vi "CheesyDrive2016Ported.vi"(9 "Is Quick Turn":bool, 10 "Wheel":dbl(slide) scale=-1.0..1.0, 11 "Throttle":dbl(slide) scale=-1.0..1.0) -> (2 "RightOutput":dbl, 3 "LeftOutput":dbl)   [LabVIEW 2018]
panel:
  in  "Alpha":dbl
  in  "Wheel Deadband":dbl
  in  "Throttle Deadband":dbl
  in  "TurnSensitivity":dbl
  # "Direct Port to Labveiw from https://github.com/Team254/FRC-2016-Public/blob/master/src/com/team254/frc2016/CheesyDriveHelper.java"
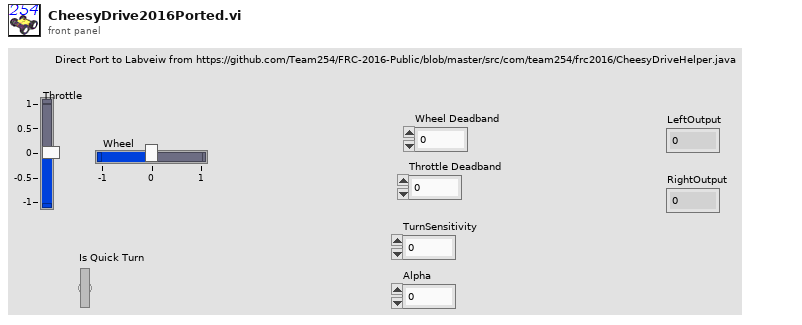
[diagram p1: front panel]
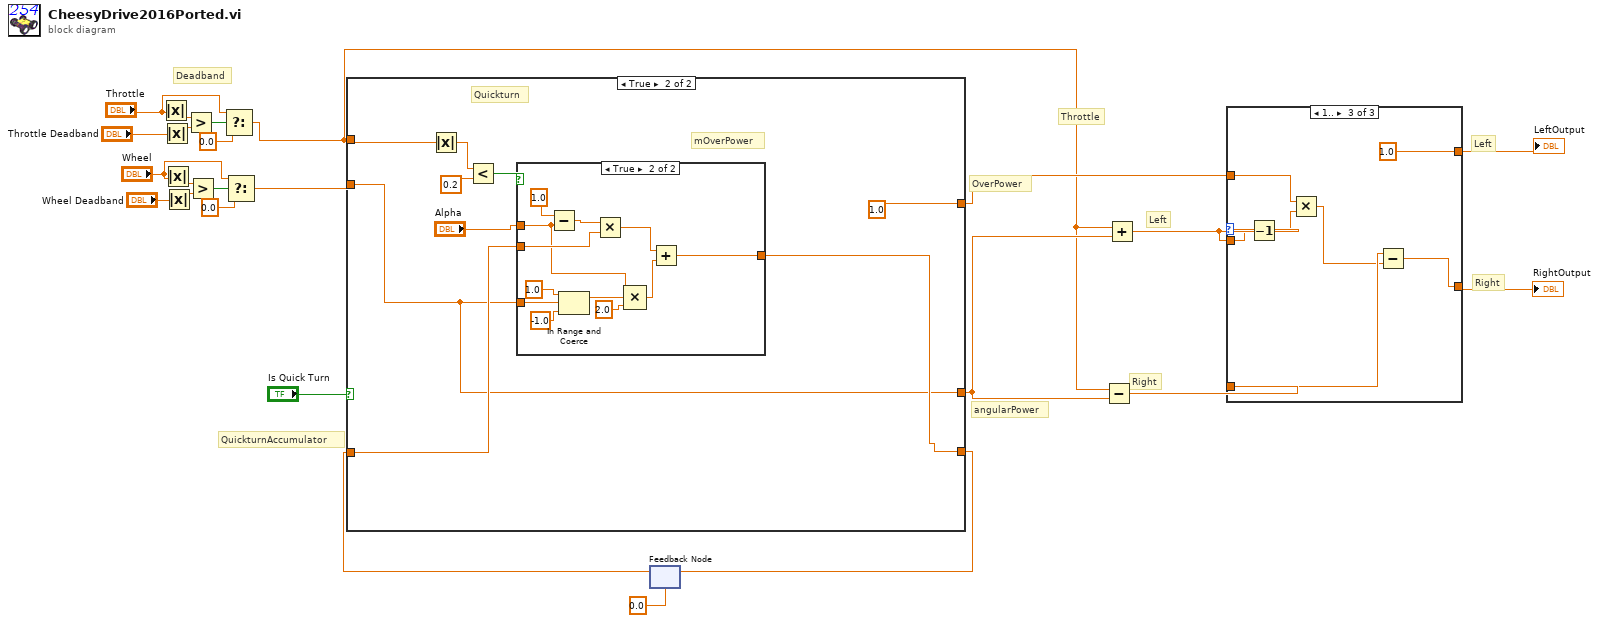
[diagram p0: block diagram]
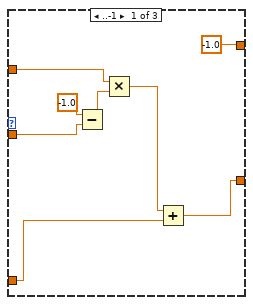
[diagram p2: hidden frame]
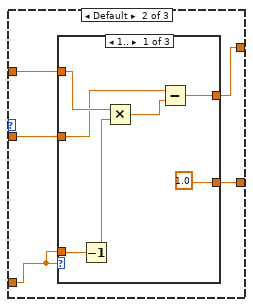
[diagram p3: hidden frame]
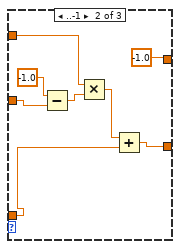
[diagram p4: hidden frame]
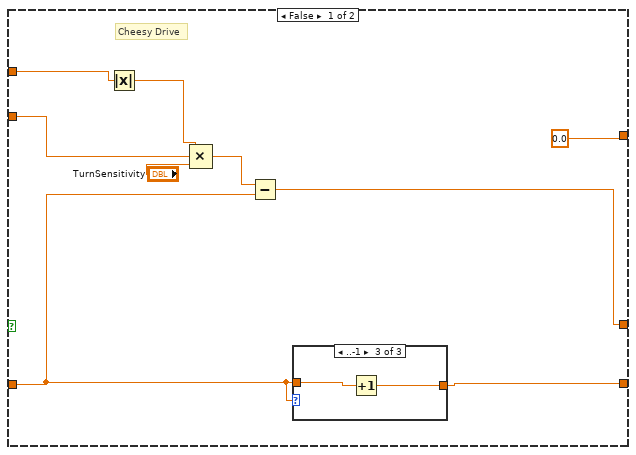
[diagram p6: hidden frame]
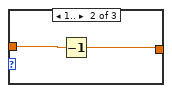
[diagram p8: hidden frame]
diagram:
  # "Deadband"
  # "Right"
  # "Left"
  # "Throttle"
  # "Left"
  # "Right"
  # "QuickturnAccumulator"
  # "angularPower"
  # "OverPower"
  n1 = Absolute Value(x="Throttle") -> (abs(x)=w15:dbl)
  n2 = Absolute Value(x="Throttle Deadband") -> (abs(x)=w14:dbl)
  n3 = Absolute Value(x="Wheel") -> (abs(x)=w10:dbl)
  n4 = Absolute Value(x="Wheel Deadband") -> (abs(x)=w11:dbl)
  n5 = Greater?(x=w15, y=w14) -> (0:w16:bool)
  n6 = Greater?(x=w10, y=w11) -> (0:w9:bool)
  n7 = Select(t="Throttle", s=w16, f=0.0) -> (s? t:f=w7:dbl)
  n8 = Select(t="Wheel", s=w9, f=0.0) -> (s? t:f=w8:dbl)
  n9 = feedback #1(0.0) -> (w22:dbl)
  n10 = case shown="True" "Is Quick Turn" {
    tunnel: w7 -> [w33 w47]
    tunnel: w8 -> [w31 w40]
    tunnel: [w26 w42] -> w23
    tunnel: w22 -> [w27 w43]
    tunnel: [0.0 1.0] -> w19
    tunnel: [w29 w40] -> w20
    frame False {
      # "Cheesy Drive"
      n11 = Absolute Value(x=w33) -> (abs(x)=w32:dbl)
      n12 = Compound Arithmetic op=MULTIPLY(w32, w31, "TurnSensitivity") -> (w30:dbl)
      n13 = Subtract(x=w30, y=w27) -> (x-y=w29:dbl)
      n14 = case shown="..-1" w27 {
        tunnel: w27 -> [w34 w36 w38]
        tunnel: [w34 w35 w37] -> w26
        frame Default {
        }
        frame 1.. {
          n15 = Decrement(x=w36) -> (x-1=w35:dbl)
        }
        frame ..-1 {
          n16 = Increment(x=w38) -> (x+1=w37:dbl)
        }
      }
    }
    frame True {
      # "mOverPower"
      # "Quickturn"
      n17 = Absolute Value(x=w47) -> (abs(x)=w45:dbl)
      n18 = Less?(x=w45, y=0.2) -> (x < y?=w46:bool)
      n19 = case shown="True" w46 {
        tunnel: w43 -> [w48 w59]
        tunnel: "Alpha" -> [_ w56]
        tunnel: w40 -> [_ w53]
        tunnel: [w48 w49] -> w42
        frame False {
        }
        frame True {
          n20 = Subtract(x=1.0, y=w56) -> (x-y=w60:dbl)
          n21 = In Range and Coerce(upper limit=1.0, x=w53, lower limit=-1.0) -> (coerced(x)=w54:dbl)  [unwired: 1 out]
          n22 = Multiply(x=w60, y=w59) -> (x*y=w57:dbl)
          n23 = Compound Arithmetic op=MULTIPLY(w56, w54, 2.0) -> (w50:dbl)
          n24 = Add(x=w57, y=w50) -> (x+y=w49:dbl)
        }
      }
    }
  }
  n25 = feedback-in #1(w23) -> ()
  n26 = Subtract(x=w7, y=w20) -> (x-y=w18:dbl)
  n27 = Add(x=w7, y=w20) -> (x+y=w17:dbl)
  n28 = case shown="1.." w17 {
    tunnel: [-1.0 w69 1.0] -> w2
    tunnel: w19 -> [w64 w71 w94]
    tunnel: w18 -> [w62 w73 w92]
    tunnel: [w61 w70 w93] -> w1
    tunnel: w17 -> [w66 w72 w96]
    frame ..-1 {
      n29 = Subtract(x=-1.0, y=w66) -> (x-y=w65:dbl)
      n30 = Multiply(x=w64, y=w65) -> (x*y=w63:dbl)
      n31 = Add(x=w63, y=w62) -> (x+y=w61:dbl)
    }
    frame Default {
      n32 = case shown="1.." w73 {
        tunnel: w73 -> [w79 w81 w89]
        tunnel: w72 -> [w75 w87 w90]
        tunnel: w71 -> [w78 w84 _]
        tunnel: [1.0 w83 w89] -> w70
        tunnel: [w76 -1.0 w90] -> w69
        frame 1.. {
          n33 = Decrement(x=w79) -> (x-1=w77:dbl)
          n34 = Multiply(x=w78, y=w77) -> (x*y=w74:dbl)
          n35 = Subtract(x=w75, y=w74) -> (x-y=w76:dbl)
        }
        frame ..-1 {
          n36 = Subtract(x=-1.0, y=w87) -> (x-y=w85:dbl)
          n37 = Multiply(x=w84, y=w85) -> (x*y=w82:dbl)
          n38 = Add(x=w82, y=w81) -> (x+y=w83:dbl)
        }
        frame Default {
        }
      }
    }
    frame 1.. {
      n39 = Decrement(x=w96) -> (x-1=w95:dbl)
      n40 = Multiply(x=w94, y=w95) -> (x*y=w91:dbl)
      n41 = Subtract(x=w92, y=w91) -> (x-y=w93:dbl)
    }
  }
  "LeftOutput" <- w2
  "RightOutput" <- w1
